vi "Save Values Remote.vi"(8 "error in (no error)":errorcluster, 11 "Board Game in":refnum<class "Board Game.lvclass">) -> (0 "error out":errorcluster)   [LabVIEW 2021, in "Board Game.lvclass"]
uses:
  Board Game.lvclass
  Board Game.lvclass/Board Game.ctl
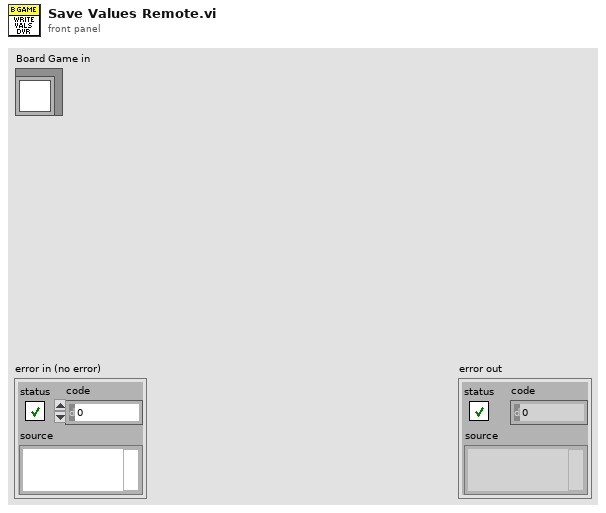
[diagram p1: front panel]
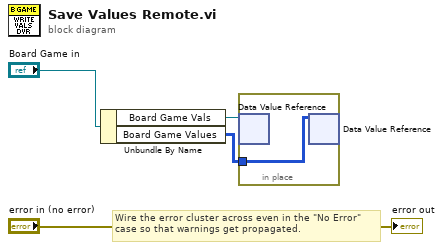
[diagram p0: block diagram]
diagram:
  # "Wire the error cluster across even in the \"No Error\"\ncase so that warnings get propagated."
  n1 = Unbundle By Name("Board Game in") -> ("Board Game Vals"=w2:refnum<data-value>, "Board Game Values"=w1:u32[][])
  n2 = in-place {
    in-place-border: w1 -> [w5]
    n3 = in-place-dvr #1(w2) -> ()  [unwired: 2 out]
    n4 = in-place-dvr #1(w5) -> ()  [unwired: 2 out]
  }
  "error out" <- "error in (no error)"
